vi "Tausand AB1000 Sleep Time Sweep Example (StateMachine).vi"() -> ()   [LabVIEW 2015]
doc: "Example of sleep time sweep for a single channel with a Tausand Abacus device.\n\nVerifies if the selected port is valid, then changes the sleep time in the given range. Measures a single time at each sleep time. Produces live graphics.\nBlock diagram coded as a state machine."
uses:
  <instrlib>/Tausand AB1000/Public/Controls/deviceTypeRing.ctl
  <instrlib>/Tausand AB1000/Public/Controls/channelRing.ctl
  <instrlib>/Tausand AB1000/Examples/sub vi/sleepTimeSweep_states.ctl
  <instrlib>/Tausand AB1000/Tausand AB1000.lvlib
panel:
  out "2ch device?":bool
  in  "Input channel":T1=1 items=["A"=1, "B"=2, "C"=3, "D"=4]
  out "device type":T2 items=["any"=0, "AB1002"=1002, "AB1004"=1004, "AB1502"=1502, "AB1504"=1504, "AB2002"=2002, "AB2004"=2004, "AB2502"=2502, "AB2504"=2504]
  out "Counts at last sleep time":u32
  out "counts array":u32[](array[numeric])
  in  "Sampling time (ms)":u32(ring)=1000 items=["1000s"=1000000, "500s"=500000, "200s"=200000, "100s"=100000, "50s"=50000, "20s"=20000, "10s"=10000, "5s"=5000, "2s"=2000, "1s"=1000, "500ms"=500, "200ms"=200, "100ms"=100, "50ms"=50, "20ms"=20, "10ms"=10, "5ms"=5, "2ms"=2, "1ms"=1]
  in  "step":i32=10 min=1 max=100 step=1
  out "progressStr":string
  out "current sleepTime":i32
  out "valid data?":bool
  out "dataID":u32
  out "Total progress":dbl(slide) scale=0.0..100.0
  out "number of sleeptimes":i32
  out "sleepTime index":i32
  out "wait done?":bool
  out "nextRead":u32 caption="next read in"
  out "current time":timestamp
  out "wait until":timestamp
  in  "stop":bool
  out "sleepTime array":i32[](array[numeric])
  out "Grph":cluster{i32[], u32[]}(graph)
  in  "Sleep time range (ns)":cluster{i32, i32}(slide)={-20, 20} scale=0.0..100.0
  out "valid device?":bool
  in  "VISA port":refnum<visa-resource-name>
  # "Overview: example doing a sleep time sweep in a single input channel with a Tausand Abacus AB1002, AB1502, AB1004, AB1504, AB2004 and AB2504 device.\nInstructions:\n1. Select the VISA port.\n2. Enter the desired settings.\n3. Run the VI.\n4. Click stop to abort the VI execution."
  # "August 2021"
  # "Set these values before running the VI."
  # "Sleep time in progess:"
  # "ns"
  # "s"
  # "from"
  # "to"
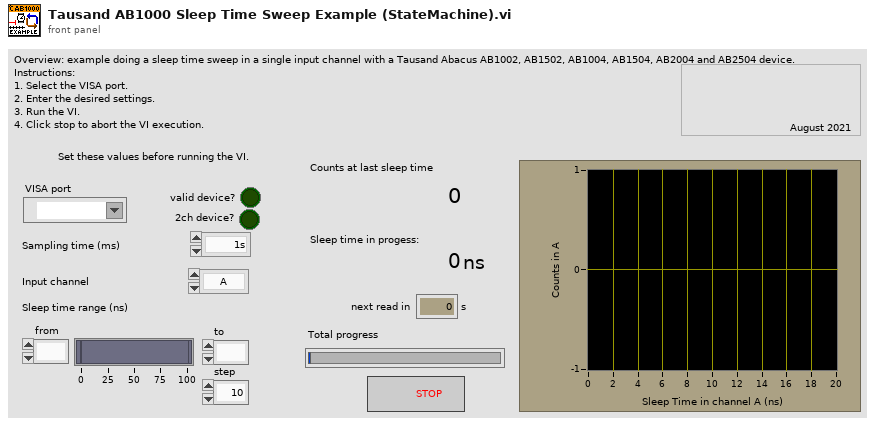
[diagram p1: front panel]
types:
  T1 = typedef "Tausand AB1000.lvlib/channelRing.ctl" = u8
  T2 = typedef "Tausand AB1000.lvlib/deviceTypeRing.ctl" = u16
  T3 = typedef "sleepTimeSweep_states.ctl" = enum16{"update sleepTime range", "create sleepTime array", "verify port", "invalid port message", "create counter array", "initialize device", "set sleepTime", "set wait timer", "wait sampling time", "read data", "graph data", "increase index", "repeat measurement", "close device", "end state"}
  T4 = typedef "Tausand AB1000.lvlib/counters4ch.ctl" = cluster{"counter_A":u32, "counter_B":u32, "counter_C":u32, "counter_D":u32, "counter_AB":u32, "counter_AC":u32, "counter_AD":u32, "counter_BC":u32, "counter_BD":u32, "counter_CD":u32, "counter_multiple_1":u32, "counters_ID":u32, "time_left":u32}
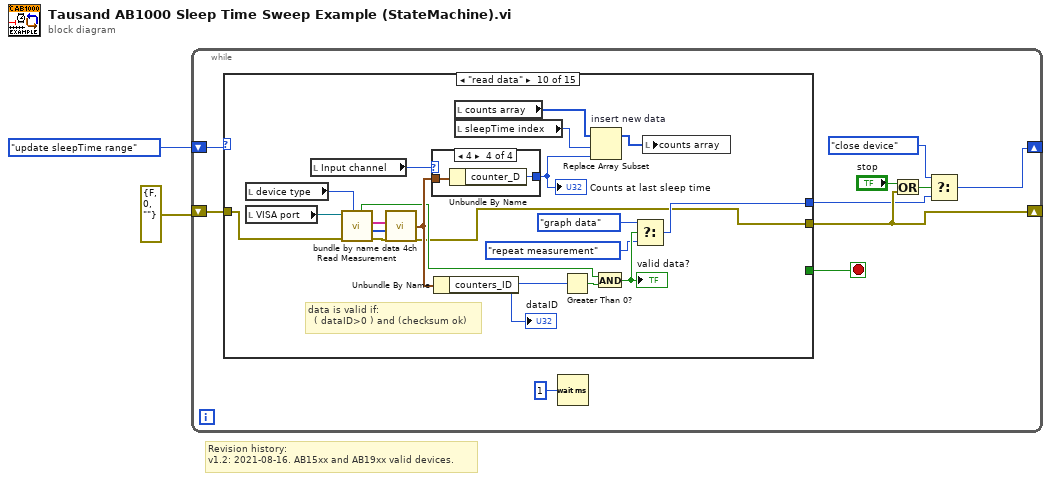
[diagram p0: block diagram]
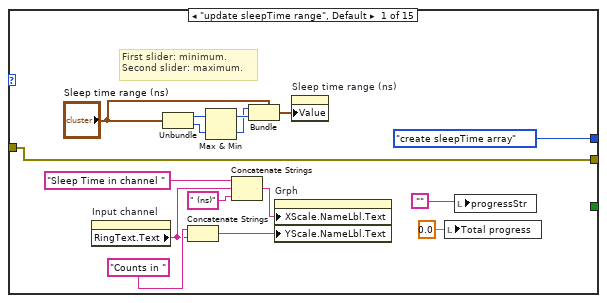
[diagram p2: hidden frame]
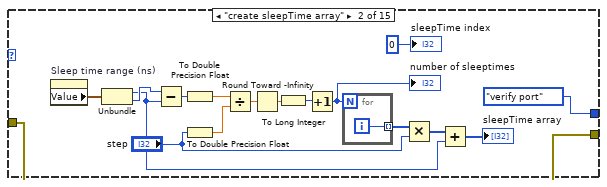
[diagram p3: hidden frame]
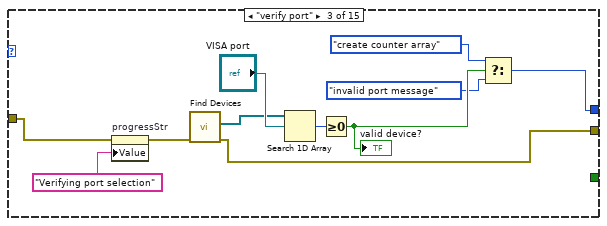
[diagram p4: hidden frame]
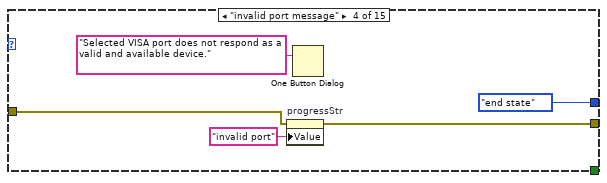
[diagram p5: hidden frame]
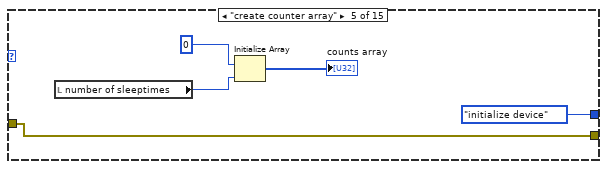
[diagram p6: hidden frame]
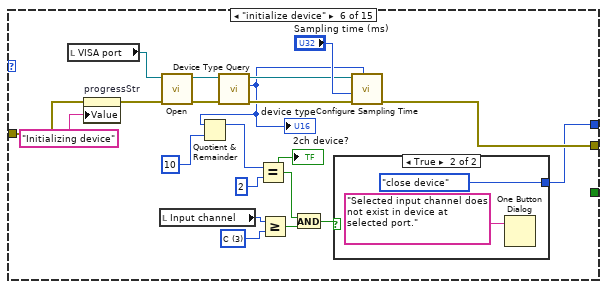
[diagram p7: hidden frame]
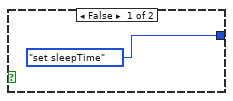
[diagram p8: hidden frame]
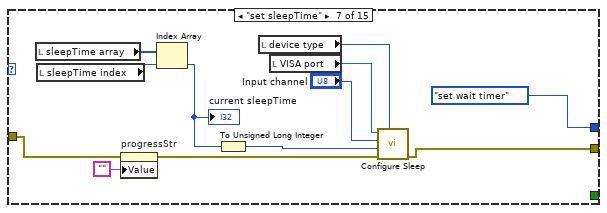
[diagram p9: hidden frame]
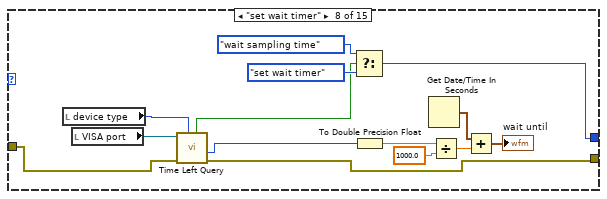
[diagram p10: hidden frame]
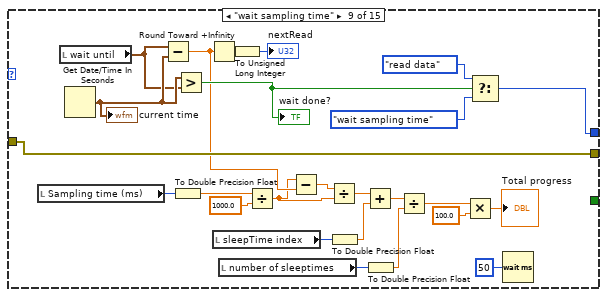
[diagram p11: hidden frame]
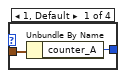
[diagram p12: hidden frame]
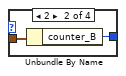
[diagram p13: hidden frame]
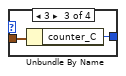
[diagram p14: hidden frame]
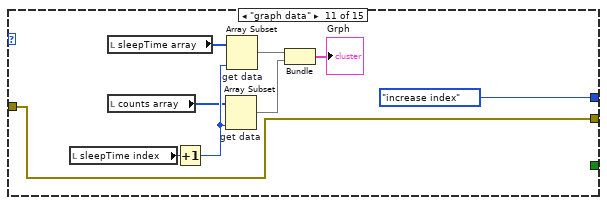
[diagram p15: hidden frame]
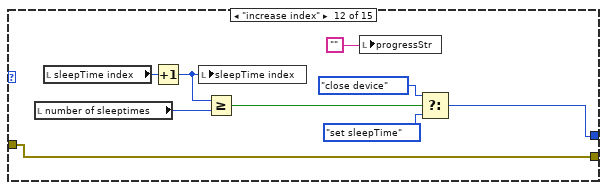
[diagram p16: hidden frame]
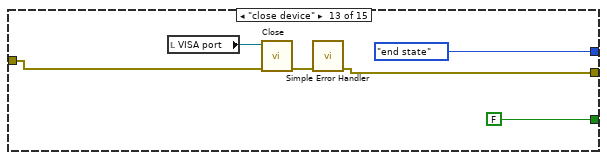
[diagram p17: hidden frame]
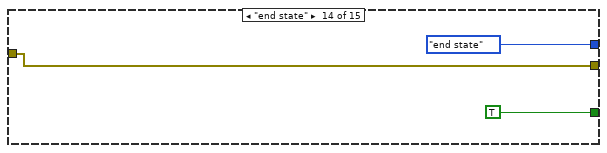
[diagram p18: hidden frame]
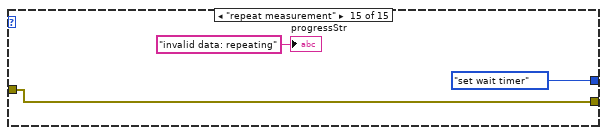
[diagram p19: hidden frame]
diagram:
  # "Revision history:\nv1.2: 2021-08-16. AB15xx and AB19xx valid devices."
  n1 = while {
    shift-right: [w4] -> _
    shift-left: sleepTimeSweep_states."update sleepTime range" ("Enum") -> [w5]
    shift-right: [w8] -> _
    shift-left: errorcluster {"status"=FALSE, "code"=0, "source"=""} ("error in (no error)") -> [w11]
    stop <- w10 stop-if-true
    n2 = case shown="\"read data\"" w5 {
      tunnel: [_ _ _ _ _ _ _ _ _ _ _ _ FALSE TRUE _] -> w10
      tunnel: w11 -> [w22 w35 w50 w60 w67 w86 w99 w104 w141 w144 w177 w186 w190 w194 w198]
      tunnel: [w22 w35 w48 w59 w67 w78 w92 w103 w141 w143 w177 w186 w189 w194 w198] -> w8
      tunnel: [sleepTimeSweep_states."create sleepTime array" sleepTimeSweep_states."verify port" w47 sleepTimeSweep_states."end state" sleepTimeSweep_states."initialize device" w72 sleepTimeSweep_states."set wait timer" w109 w121 w153 sleepTimeSweep_states."increase index" w178 sleepTimeSweep_states."end state" sleepTimeSweep_states."end state" sleepTimeSweep_states."set wait timer"] -> w3
      frame "update sleepTime range", Default {
        # "First slider: minimum.\nSecond slider: maximum."
        n3 = property on="Input channel" class="Ring (strict)"() -> ("RingText.Text"=w13:string)  [unwired: 2 in, 2 out]
        n4 = Unbundle("Sleep time range (ns)") -> (w28:i32, w24:i32)
        n5 = Concatenate Strings("Counts in ", w13) -> (w17:string)
        n6 = Max & Min(x=w28, y=w24) -> (max(x,y)=w25:i32, min(x,y)=w23:i32)
        n7 = Concatenate Strings("Sleep Time in channel ", w13, " (ns)" ("string")) -> (w14:string)
        n8 = Bundle(cluster="Sleep time range (ns)", w23, w25) -> (w26:cluster{i32, i32})
        n9 = property on="Grph" class="XYGraph (strict)"("XScale.NameLbl.Text"=w14, "YScale.NameLbl.Text"=w17) -> ()  [unwired: 2 in, 2 out]
        n10 = property on="Sleep time range (ns)" class="Slide (strict)"("Value"=w26) -> ()  [unwired: 2 in, 2 out]
        n11 = local write "Total progress"(0.0 ("Total progress")) -> ()
        n12 = local write "progressStr"("") -> ()
      }
      frame "create sleepTime array" {
        n13 = property on="Sleep time range (ns)" class="Slide (strict)"() -> ("Value"=w38:cluster{i32, i32})  [unwired: 2 in, 2 out]
        n14 = Unbundle(w38) -> (w36:i32, w37:i32)
        n15 = Subtract(x=w37, y=w36) -> (x-y=w45:i32)
        n16 = To Double Precision Float(number=w45) -> (double precision float=w43:dbl)
        n17 = To Double Precision Float(number="step") -> (double precision float=w42:dbl)
        n18 = Divide(x=w43, y=w42) -> (x/y=w31:dbl)
        n19 = Round Toward -Infinity(1:w31) -> (0:w30:dbl)
        n20 = To Long Integer(number=w30) -> (32bit integer=w39:i32)
        n21 = Increment(x=w39) -> (x+1=w32:i32)
        "number of sleeptimes" <- w32
        n22 = for {
          N: w32 -> [_]
          tunnel: [w46] -> w44 mode=indexing
          i -> [w46]
        }
        n23 = Multiply(x=w44, y="step") -> (x*y=w40:i32[])
        n24 = Add(x=w40, y=w36) -> (x+y=→"sleepTime array":i32[])
        "sleepTime index" <- 0 ("delay index")
      }
      frame "verify port" {
        n25 = property on="progressStr" class="Str"(error in=w50, "Value"="Verifying port selection" ("progressStr")) -> (error out=w49:errorcluster)  [unwired: 1 in, 1 out]
        n26 = call <instrlib>:"Find Devices.vi"("error in (no error)"=w49) -> ("error out"=w48:errorcluster, "Abacus VISAs"=w55:refnum<visa-resource-name>[])  [unwired: 8 in, 1 out]
        n27 = Search 1D Array(1D array=w55, element="VISA port") -> (index of element=w57:i32)  [unwired: 1 in]
        n28 = Greater Or Equal To 0?(x=w57) -> (x >= 0?=w54:bool)
        "valid device?" <- w54
        n29 = Select(t=sleepTimeSweep_states."create counter array", s=w54, f=sleepTimeSweep_states."invalid port message") -> (s? t:f=w47:T3)
      }
      frame "invalid port message" {
        n30 = property on="progressStr" class="Str"(error in=w60, "Value"="invalid port" ("progressStr")) -> (error out=w59:errorcluster)  [unwired: 1 in, 1 out]
        n31 = One Button Dialog(message="Selected VISA port does not respond as a valid and available device.") -> ()  [unwired: 1 in, 1 out]
      }
      frame "create counter array" {
        n32 = local read "number of sleeptimes"() -> (w66:i32)
        n33 = Initialize Array "Initialize Array"(u32 0 ("counts"), w66) -> (→"counts array":u32[])
      }
      frame "initialize device" {
        w76 = T1 3 items=["none", "A", "B", "C", "D", "E", "F", "G", "H"] ("Input channel")
        n34 = local read "VISA port"() -> (w84:refnum<visa-resource-name>)
        n35 = property on="progressStr" class="Str"(error in=w86, "Value"="Initializing device" ("progressStr")) -> (error out=w85:errorcluster)  [unwired: 1 in, 1 out]
        n36 = local read "Input channel"() -> (w77:T1)
        n37 = call <instrlib>:"Open.vi"("error in (no error)"=w85, "VISA resource name"=w84) -> ("error out"=w83:errorcluster, "VISA resource name out"=w82:refnum<visa-resource-name>)  [unwired: 8 in]
        n38 = call <instrlib>:"Device Type Query.vi"("error in (no error)"=w83, "VISA Refnum in"=w82) -> ("error out"=w79:errorcluster, "device type"=w68:T2, "VISA Refnum out"=w80:refnum<visa-resource-name>)  [unwired: 7 in]
        "device type" <- w68
        n39 = Quotient & Remainder(x=w68, y=u16 10 ("Numeric")) -> (x-y*floor(x/y)=w70:T2)  [unwired: 1 out]
        n40 = Equal?(x=w70, y=u16 2 ("Numeric")) -> (x = y?=w74:bool)
        "2ch device?" <- w74
        n41 = Greater Or Equal?(x=w77, y=w76) -> (x >= y?=w75:bool)
        n42 = And(x=w74, y=w75) -> (x .and. y?=w73:bool)
        n43 = case shown="True" w73 {
          tunnel: [sleepTimeSweep_states."set sleepTime" sleepTimeSweep_states."close device"] -> w72
          frame False {
          }
          frame True {
            n44 = One Button Dialog(message="Selected input channel does not exist in device at selected port.") -> ()  [unwired: 1 in, 1 out]
          }
        }
        n45 = call <instrlib>:"Configure Sampling Time.vi"("device type"=w68, "error in (no error)"=w79, "value (1000 ms)"="Sampling time (ms)", "VISA Refnum in"=w80) -> ("error out"=w78:errorcluster)  [unwired: 5 in, 2 out]
      }
      frame "set sleepTime" {
        n46 = local read "sleepTime array"() -> (w102:i32[])
        n47 = local read "sleepTime index"() -> (w101:i32)
        n48 = property on="progressStr" class="Str"(error in=w99, "Value"="" ("progressStr")) -> (error out=w93:errorcluster)  [unwired: 1 in, 1 out]
        n49 = Index Array(array=w102, index=w101) -> (element=w97:i32)
        "current sleepTime" <- w97
        n50 = To Unsigned Long Integer(number=w97) -> (unsigned 32bit integer=w94:u32)
        n51 = local read "device type"() -> (w95:T2)
        n52 = local read "VISA port"() -> (w96:refnum<visa-resource-name>)
        n53 = call <instrlib>:"Configure Sleep.vi"("device type"=w95, "error in (no error)"=w93, "value (0 ns)"=w94, "channel"="Input channel", "VISA Refnum in"=w96) -> ("error out"=w92:errorcluster)  [unwired: 4 in, 2 out]
      }
      frame "set wait timer" {
        n54 = local read "device type"() -> (w107:T2)
        n55 = local read "VISA port"() -> (w108:refnum<visa-resource-name>)
        n56 = call <instrlib>:"Time Left Query.vi"("device type"=w107, "error in (no error)"=w104, "VISA Refnum in"=w108) -> ("error out"=w103:errorcluster, "time left ms out"=w106:u32, "checksum ok?"=w105:bool)  [unwired: 5 in, 1 out]
        n57 = Select(t=sleepTimeSweep_states."wait sampling time", s=w105, f=sleepTimeSweep_states."set wait timer") -> (s? t:f=w109:T3)
        n58 = To Double Precision Float(number=w106) -> (double precision float=w112:dbl)
        n59 = Get Date/Time In Seconds() -> (seconds since 1Jan1904=w115:timestamp)
        n60 = Divide(x=w112, y=1000.0) -> (x/y=w113:dbl)
        n61 = Add(x=w115, y=w113) -> (x+y=→"wait until":timestamp)
      }
      frame "wait sampling time" {
        n62 = local read "Sampling time (ms)"() -> (w118:u32)
        n63 = local read "wait until"() -> (w139:timestamp)
        n64 = Get Date/Time In Seconds() -> (seconds since 1Jan1904=w140:timestamp)
        "current time" <- w140
        n65 = Subtract(x=w139, y=w140) -> (x-y=w129:dbl)
        n66 = To Double Precision Float(number=w118) -> (double precision float=w119:dbl)
        n67 = Greater?(x=w140, y=w139) -> (0:w136:bool)
        "wait done?" <- w136
        n68 = Round Toward +Infinity(x=w129) -> (ceil(x): smallest int >= x=w138:dbl)
        n69 = local read "sleepTime index"() -> (w125:i32)
        n70 = local read "number of sleeptimes"() -> (w126:i32)
        n71 = To Unsigned Long Integer(number=w138) -> (unsigned 32bit integer=→"nextRead":u32)
        n72 = Divide(x=w119, y=1000.0) -> (x/y=w117:dbl)
        n73 = Subtract(x=w117, y=w129) -> (x-y=w128:dbl)
        n74 = Divide(x=w128, y=w117) -> (x/y=w127:dbl)
        n75 = To Double Precision Float(number=w125) -> (double precision float=w124:dbl)
        n76 = Add(x=w127, y=w124) -> (x+y=w130:dbl)
        n77 = To Double Precision Float(number=w126) -> (double precision float=w122:dbl)
        n78 = Divide(x=w130, y=w122) -> (x/y=w132:dbl)
        n79 = Multiply(x=w132, y=100.0) -> (x*y=→"Total progress":dbl)
        n80 = Select(t=sleepTimeSweep_states."read data", s=w136, f=sleepTimeSweep_states."wait sampling time") -> (s? t:f=w121:T3)
        n81 = Wait (ms)(milliseconds to wait=u32 50) -> ()  [unwired: 1 out]
      }
      frame "read data" {
        # "data is valid if:\n  ( dataID>0 ) and (checksum ok)"
        n82 = local read "device type"() -> (w142:T2)
        n83 = local read "VISA port"() -> (w149:refnum<visa-resource-name>)
        n84 = local read "Input channel"() -> (w151:T1)
        n85 = call <instrlib>:"Read Measurement.vi"("device type"=w142, "error in (no error)"=w144, "VISA Refnum in"=w149) -> ("error out"=w143:errorcluster, "values"=w147:u32[], "labels"=w148:string[], "checksum ok?"=w145:bool)  [unwired: 3 in, 2 out]
        n86 = call <instrlib>:"bundle by name data 4ch.vi"("names"=w148, "values"=w147) -> ("output cluster 4ch"=w146:T4)  [unwired: 13 in]
        n87 = case shown="4" w151 {
          tunnel: [w162 w164 w166 w168] -> w152
          tunnel: w146 -> [w161 w163 w165 w167]
          frame 1, Default {
            n88 = Unbundle By Name(w161) -> ("counter_A"=w162:u32)
          }
          frame 2 {
            n89 = Unbundle By Name(w163) -> ("counter_B"=w164:u32)
          }
          frame 3 {
            n90 = Unbundle By Name(w165) -> ("counter_C"=w166:u32)
          }
          frame 4 {
            n91 = Unbundle By Name(w167) -> ("counter_D"=w168:u32)
          }
        }
        "Counts at last sleep time" <- w152
        n92 = Unbundle By Name(w146) -> ("counters_ID"=w150:u32)
        "dataID" <- w150
        n93 = local read "counts array"() -> (w159:u32[])
        n94 = local read "sleepTime index"() -> (w158:i32)
        n95 = Greater Than 0?(x=w150) -> (x > 0?=w157:bool)
        n96 = Replace Array Subset "insert new data"(array=w159, new element=w152, index=w158) -> (w160:u32[])
        n97 = And(x=w145, y=w157) -> (x .and. y?=w156:bool)
        "valid data?" <- w156
        n98 = Select(t=sleepTimeSweep_states."graph data", s=w156, f=sleepTimeSweep_states."repeat measurement") -> (s? t:f=w153:T3)
        n99 = local write "counts array"(w160) -> ()
      }
      frame "graph data" {
        n100 = local read "sleepTime index"() -> (w174:i32)
        n101 = local read "sleepTime array"() -> (w175:i32[])
        n102 = local read "counts array"() -> (w171:u32[])
        n103 = Increment(x=w174) -> (x+1=w173:i32)
        n104 = Array Subset "get data"(array=w171, length=w173) -> (w170:u32[])  [unwired: 1 in]
        n105 = Array Subset "get data"(array=w175, length=w173) -> (w176:i32[])  [unwired: 1 in]
        n106 = Bundle(w176, w170) -> (→"Grph":cluster{i32[], u32[]})  [unwired: 1 in]
      }
      frame "increase index" {
        n107 = local read "number of sleeptimes"() -> (w183:i32)
        n108 = local read "sleepTime index"() -> (w185:i32)
        n109 = Increment(x=w185) -> (x+1=w184:i32)
        n110 = local write "sleepTime index"(w184) -> ()
        n111 = Greater Or Equal?(x=w184, y=w183) -> (x >= y?=w182:bool)
        n112 = local write "progressStr"("") -> ()
        n113 = Select(t=sleepTimeSweep_states."close device", s=w182, f=sleepTimeSweep_states."set sleepTime") -> (s? t:f=w178:T3)
      }
      frame "close device" {
        n114 = local read "VISA port"() -> (w188:refnum<visa-resource-name>)
        n115 = call <instrlib>:"Close.vi"("error in (no error)"=w190, "VISA resource name"=w188) -> ("error out"=w191:errorcluster)  [unwired: 9 in]
        n116 = call <vilib>:"Simple Error Handler.vi"("error in (no error)"=w191) -> ("error out"=w189:errorcluster)  [unwired: 4 in, 4 out]
      }
      frame "end state" {
      }
      frame "repeat measurement" {
        "progressStr" <- "invalid data: repeating" ("repeatingStr")
      }
    }
    n117 = Wait (ms)(milliseconds to wait=u32 1) -> ()  [unwired: 1 out]
    n118 = Or(x="stop", y=w8) -> (x .or. y?=w6:bool)
    n119 = Select(t=sleepTimeSweep_states."close device", s=w6, f=w3) -> (s? t:f=w4:T3)
  }
